vi "FG COP Waypoints.vi"(1 "FG Action (Read)":T1, 2 "COP Waypoints in":T2) -> (0 "COP Waypoints out":T2)   [LabVIEW 2011]
uses:
  Support Files/RequestIDRec.ctl
  Support Files/ElementRec.ctl
  Support Files/LocalWaypointRec.ctl
  cRIO/Functional Global Variables/Actions for FG's.ctl
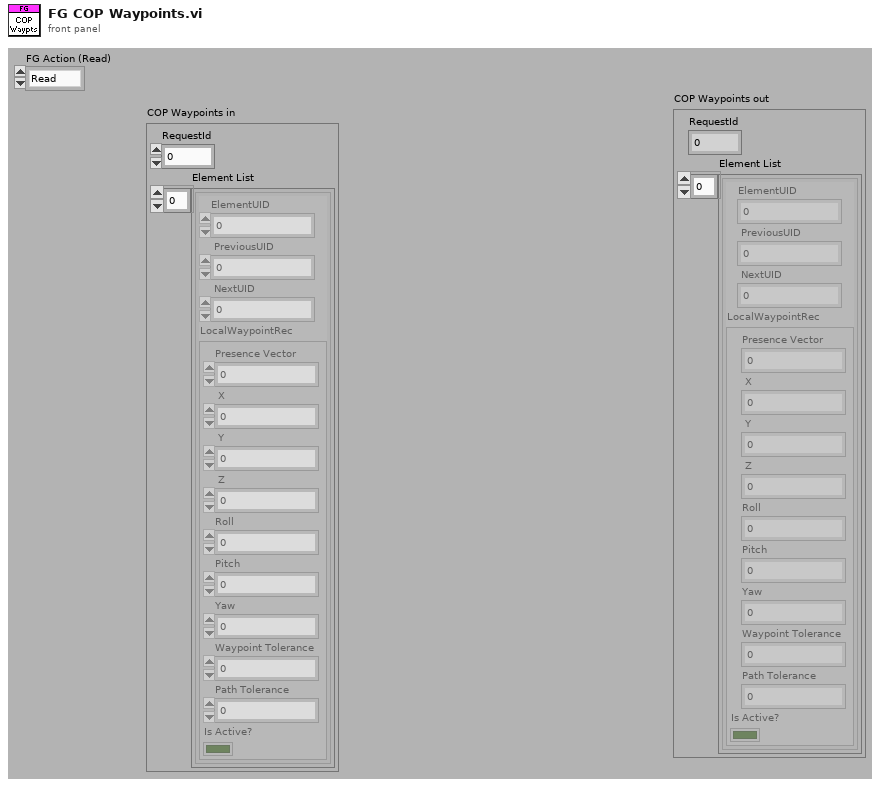
[diagram p1: front panel]
types:
  T1 = typedef "Actions for FG's.ctl" = enum16{"Read", "Write"}
  T2 = typedef "RequestIDRec.ctl" = cluster{"RequestId":u8, "Element List":T3[]}
  T3 = typedef "ElementRec.ctl" = cluster{"ElementUID":u16, " PreviousUID":u16, " NextUID":u16, "LocalWaypointRec":T4}
  T4 = typedef "LocalWaypointRec.ctl" = cluster{"Presence Vector":u8, " X":dbl, " Y":dbl, " Z":dbl, "Roll":dbl, "Pitch":dbl, "Yaw":dbl, "Waypoint Tolerance":dbl, "Path Tolerance":dbl, "Is Active?":bool}
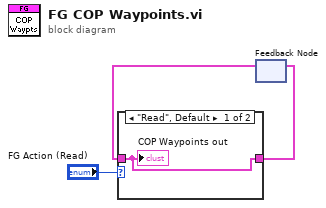
[diagram p0: block diagram]
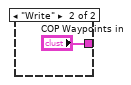
[diagram p2: hidden frame]
diagram:
  n1 = feedback #1() -> (w1:T2)  [unwired: 1 in]
  n2 = case shown="\"Read\", Default" "FG Action (Read)" {
    tunnel: w1 -> [w4 _]
    tunnel: [w4 "COP Waypoints in"] -> w2
    frame "Read", Default {
      "COP Waypoints out" <- w4
    }
    frame "Write" {
    }
  }
  n3 = feedback-in #1(w2) -> ()
